vi "Reset Encoders.vi"() -> (3 "Done?":bool)   [LabVIEW 2016]
uses:
  Robot Global Reference.vi
  Robot Values.vi
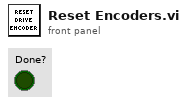
[diagram p1: front panel]
types:
  T1 = typedef "Global References.ctl" = cluster{"Joystick Reference":T2, "Drive Reference":T5, "Sensor Reference":T13, "Acquisition Reference":T20, "Shoot Reference":T21, "Gear Reference":T22, "Climb Reference":T25, "Relay Reference":cluster{"LED Ring Light":T26}}
  T2 = typedef "Joystick Reference.ctl" = cluster{"Driver Joystick":T3, "Operator Joystick":T3}
  T3 = typedef "WPI_JoystickDevRef.ctl" = cluster{"Device":T4}
  T4 = typedef "WPI_JoystickDeviceEnum.ctl" = enum16{"USB 0", "USB 1", "USB 2", "USB 3", "USB 4", "USB 5"}
  T5 = typedef "Drive Reference.ctl" = cluster{"RobotDriveDevRef":T6, "Drive PTO Solenoid":T11}
  T6 = typedef "WPI_RobotDriveDevRef.ctl" = cluster{"DevStatus":errorcluster, "Motors[]":T7[], "Square Inputs":bool, "Max Output":dbl}
  T7 = typedef "WPI_MotorControlDeviceRef.ctl" = cluster{"DeviceStatus":errorcluster, "Type":T8, "PWM":cluster{"PWM Channel":T9, "DeadBand":T10}, "CAN":cluster{"Device Number":u8, "SetOutput VI Ref":variant, "GetOutput VI Ref":variant, "Enable VI Ref":variant, "Disable VI Ref":variant, "Data":variant}, "Invert":bool}
  T8 = typedef "WPI_MotorControlType.ctl" = enum16{"PWM", "CAN"}
  T9 = typedef "FPGA_DIOPWMChannel.ctl" = enum8{"PWM 0", "PWM 1", "PWM 2", "PWM 3", "PWM 4", "PWM 5", "PWM 6", "PWM 7", "PWM 8", "PWM 9", "PWM MXP 0", "PWM MXP 1", "PWM MXP 2", "PWM MXP 3", "PWM MXP 4", "PWM MXP 5", "PWM MXP 6", "PWM MXP 7", "PWM MXP 8", "PWM MXP 9", "Invalid"}
  T10 = typedef "WPI_PWMDeadband.ctl" = cluster{"Name":string, "maxPositivePwm":i32, "minPositivePwm":i32, "centerPwm":i32, "maxNegativePwm":i32, "minNegativePwm":i32, "angularRange":u16}
  T11 = typedef "WPI_SolenoidDevRef.ctl" = cluster{"DevStatus":errorcluster, "Pneumatics Control Module":u8, "Forward Solenoid Channel":T12, "Reverse Solenoid Channel":T12}
  T12 = typedef "WPI_SolenoidChannel.ctl" = enum8{"Solenoid 0", "Solenoid 1", "Solenoid 2", "Solenoid 3", "Solenoid 4", "Solenoid 5", "Solenoid 6", "Solenoid 7", "Invalid"}
  T13 = typedef "Sensor Reference.ctl" = cluster{"LeftMotorEncoderRef":T14, "RightMotorEncoderRef":T14, "I2C Gyro":T18, "Left Shooter Wheel Encoder":T14, "Right Shooter Wheel Encoder":T14}
  T14 = typedef "WPI_EncoderDevRef.ctl" = cluster{"DevStatus":errorcluster, "EncoderIndex":T15, "CounterIndex":T16, "DistancePerCount":dbl, "Decoding Type":T17}
  T15 = typedef "FPGA_EncoderIdx.ctl" = enum8{"Enc 0", "Enc 1", "Enc 2", "Enc 3", "Enc 4", "Enc 5", "Enc 6", "Enc 7", "Invalid"}
  T16 = typedef "FPGA_CounterCtrSystemIndex.ctl" = enum8{"Ctr 0", "Ctr 1", "Ctr 2", "Ctr 3", "Ctr 4", "Ctr 5", "Ctr 6", "Ctr 7", "Invalid"}
  T17 = typedef "WPI_EncoderType.ctl" = enum16{"1x", "2x", "4x"}
  T18 = typedef "WPI_I2CDevRef.ctl" = cluster{"DevStatus":errorcluster, "Device Address":u8, "Handle":i32, "I2C Bus":T19}
  T19 = typedef "i2c_bus.ctl" = enum16{"I2C On-Board", "I2C MXP", "Invalid"}
  T20 = typedef "Acquisition Reference.ctl" = cluster{"Acquisition Conveyor Motor DevRef":T7, "Hopper Beater Bar Motor DevRef":T7}
  T21 = typedef "Shoot Reference.ctl" = cluster{"Shooter Wheel Left":T7, "Shooter Wheel Right":T7}
  T22 = typedef "Gear Reference.ctl" = cluster{"Gear Ejection Cylinder":T11, "Door Ejection Cylinder":T11, "Gear Photoeye":T23}
  T23 = typedef "WPI_DigitalInputDevRef.ctl" = cluster{"DevStatus":errorcluster, "DIO Channel":T24}
  T24 = typedef "FPGA_DIOChannel.ctl" = enum8{"DIO 0", "DIO 1", "DIO 2", "DIO 3", "DIO 4", "DIO 5", "DIO 6", "DIO 7", "DIO 8", "DIO 9", "DIO MXP 0", "DIO MXP 1", "DIO MXP 2", "DIO MXP 3", "DIO MXP 4", "DIO MXP 5", "DIO MXP 6", "DIO MXP 7", "DIO MXP 8", "DIO MXP 9", "DIO MXP 10", "DIO MXP 11", "DIO MXP 12", "DIO MXP 13", "DIO MXP 14", "DIO MXP 15", "SPI Port CS1", "SPI Port CS2", "SPI Port CS3", "SPI Port MISO", "SPI Port MOSI", "Invalid"}
  T25 = typedef "Climb Reference.ctl" = cluster{"This is a\nplaceholder,\nadd references\nas needed.":bool}
  T26 = typedef "WPI_RelayDevRef.ctl" = cluster{"DevStatus":errorcluster, "Relay Channel":T27, "Relay Direction":T28}
  T27 = typedef "FPGA_DIORelayChannel.ctl" = enum8{"Relay 0", "Relay 1", "Relay 2", "Relay 3", "Invalid"}
  T28 = typedef "WPI_RelayDirection.ctl" = enum16{"Both directions", "Forward only", "Reverse only"}
  T29 = typedef "Robot Values.ctl" = cluster{"Robot Drive":cluster{"Left Motor Power":dbl, "Right Motor Power":dbl, "Left Encoder Value":dbl, "Right Encoder Value":dbl, "High Gear?":bool, "PTO?":bool}, "Sensors":cluster{"Gyro Angle":dbl, "Recalibrate Gyro":bool, "Reset Gyro":bool}, "Climbing":cluster{"Climber State":bool, "Gear State":dbl}, "Shooter":cluster{"Shooter Wheels":bool, "Prep Wheels":bool, "Shoot":bool, "Left Shooter Wheel Speed":dbl, "Right Shooter Wheel Speed":dbl}, "Conveyor":cluster{"Conveyor State":bool}, "Robot States":cluster{"Drive mode":string, "Alliance":T30, "Position":T31}, "Gear":cluster{"Ejection Active":bool}}
  T30 = typedef "WPI_DriverStationAllianceInfo.ctl" = enum16{"Red", "Blue", "Invalid"}
  T31 = typedef "WPI_DriverStationPositionInfo.ctl" = enum16{"1", "2", "3"}
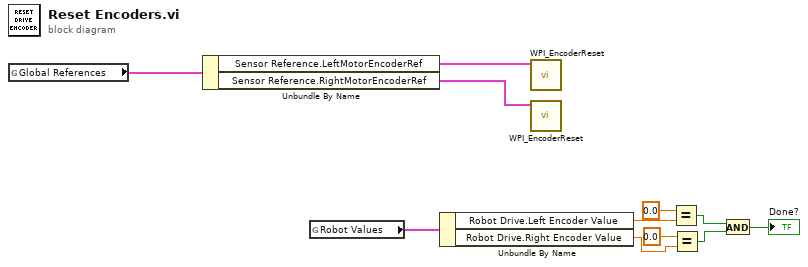
[diagram p0: block diagram]
diagram:
  n1 = global read "Robot Global Reference.vi" "Global References"() -> (w11:T1)
  n2 = Unbundle By Name(w11) -> ("Sensor Reference.LeftMotorEncoderRef"=w10:T14, "Sensor Reference.RightMotorEncoderRef"=w9:T14)
  n3 = global read "Robot Values.vi" "Robot Values"() -> (w8:T29)
  n4 = Unbundle By Name(w8) -> ("Robot Drive.Left Encoder Value"=w6:dbl, "Robot Drive.Right Encoder Value"=w5:dbl)
  n5 = call <vilib>:"WPI_EncoderReset.vi"("EncoderDevRef"=w10) -> ()  [unwired: 9 in, 2 out]
  n6 = call <vilib>:"WPI_EncoderReset.vi"("EncoderDevRef"=w9) -> ()  [unwired: 9 in, 2 out]
  n7 = Equal?(x=0.0, y=w6) -> (x = y?=w3:bool)
  n8 = Equal?(x=0.0, y=w5) -> (x = y?=w2:bool)
  n9 = And(x=w3, y=w2) -> (x .and. y?=→"Done?":bool)
